vi "Handle Errors.vi"(8 "error in (no error)":errorcluster, 10 "Location":string, 11 "Async Action In":refnum<class "Async Action.lvclass">) -> (0 "error out":errorcluster, 3 "Async Action Out":refnum<class "Async Action.lvclass">)   [LabVIEW 2020, in "Async Action.lvclass"]
uses:
  Async Action.lvclass
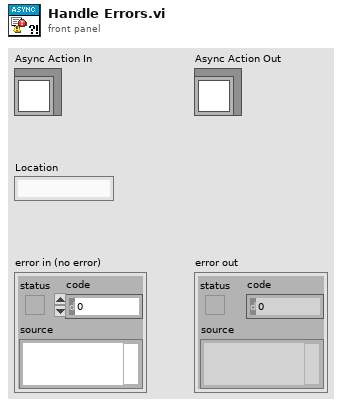
[diagram p1: front panel]
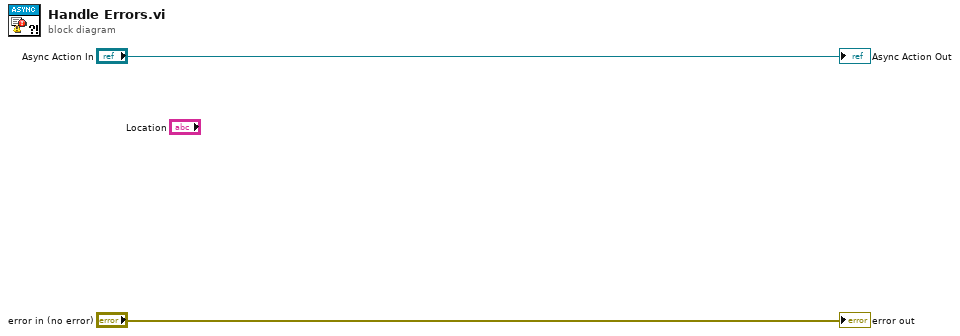
[diagram p0: block diagram]
diagram:
  "error out" <- "error in (no error)"
  "Async Action Out" <- "Async Action In"
